vi "ID MDP RAZDTC.vi"(8 "errin":errorcluster) -> (0 "errout":errorcluster, 1 "snif can":string, 2 "Messout 3":T1 {"ID" format="%x"; "MSGTYPE" format="%.0x"; "LEN" format="%.0x"; "DATA[0]" format="%.0x"; "DATA[1]" format="%.0x"; "DATA[2]" format="%.0x"; "DATA[3]" format="%.0x"; "DATA[4]" format="%.0x"; "DATA[5]" format="%.0x"; "DATA[6]" format="%.0x"; "DATA[7]" format="%.0x"}, 3 "MSG":string)   [LabVIEW 2020]
uses:
  C/Program Files (x86)/National Instruments/LabVIEW 2020/user.lib/PCAN Basic/Controls/Channel.ctl
  C/Program Files (x86)/National Instruments/LabVIEW 2020/user.lib/PCAN Basic/Controls/BaudrateEenum.ctl
  C/Program Files (x86)/National Instruments/LabVIEW 2020/user.lib/PCAN Basic/PCANBasic.lvlib
  FGV.ctl
  C/Program Files (x86)/National Instruments/LabVIEW 2020/user.lib/Alex_Peak_lib/PEAK_lib_ALEX.lvlib
panel:
  out "EXIT":bool
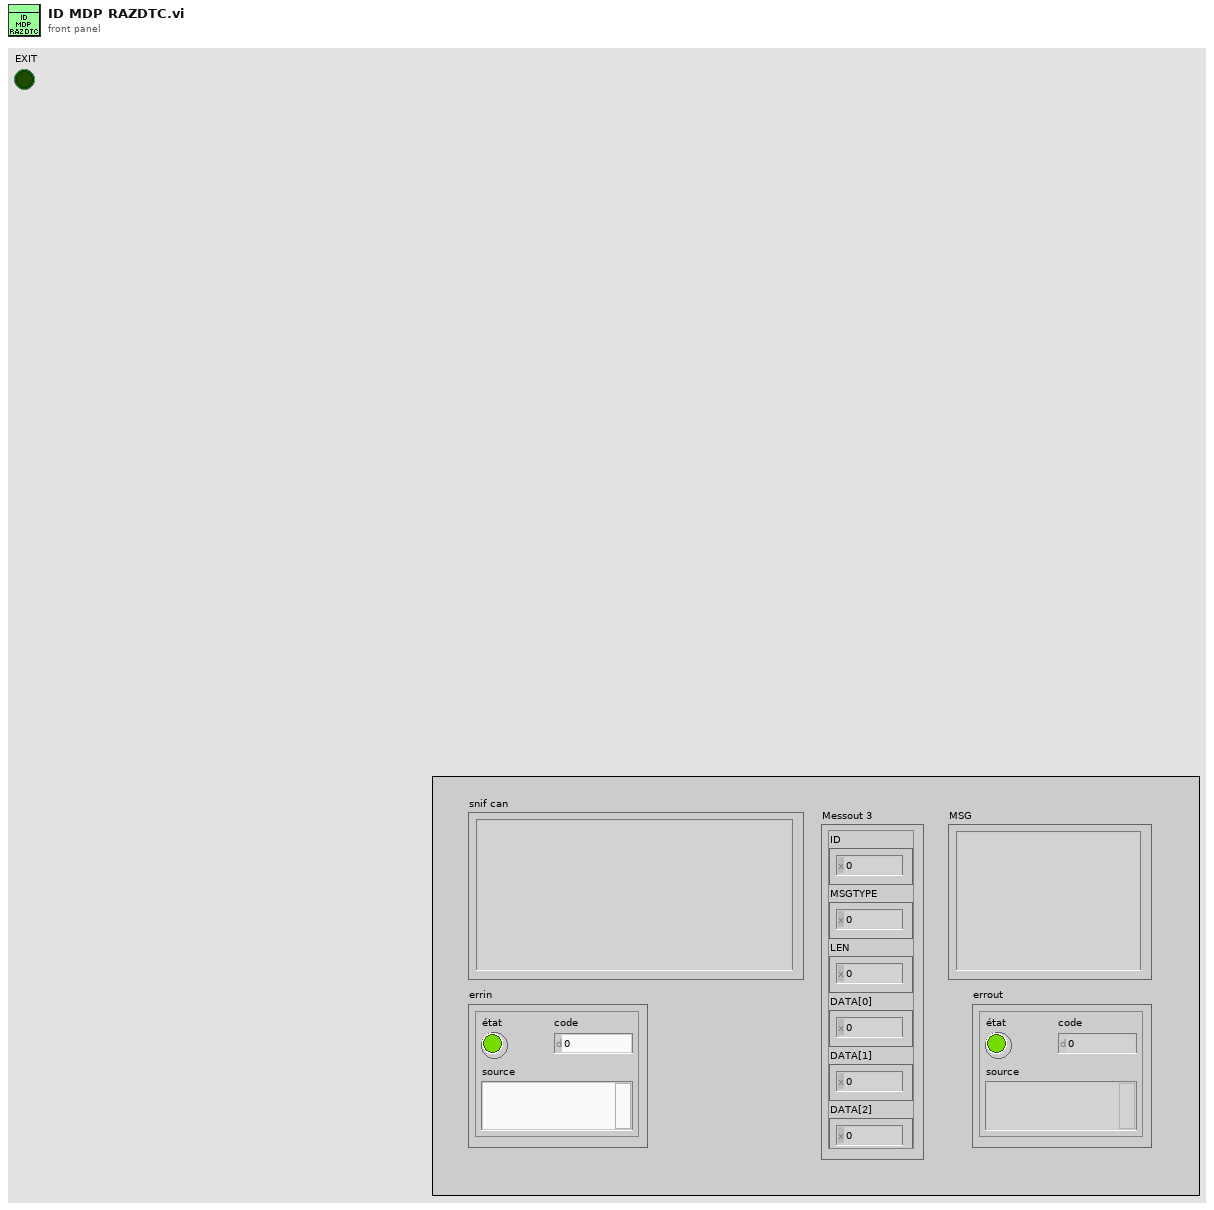
[diagram p1: front panel]
types:
  T1 = cluster{"ID":u32, "MSGTYPE":u8, "LEN":u8, "DATA[0]":u8, "DATA[1]":u8, "DATA[2]":u8, "DATA[3]":u8, "DATA[4]":u8, "DATA[5]":u8, "DATA[6]":u8, "DATA[7]":u8}
  T2 = typedef "PCANBasic.lvlib/BaudrateEenum.ctl" = enum16{"CAN_Baud_1M", "CAN_Baud_800K", "CAN_BAUD_500K", "CAN_BAUD_250K", "CAN_BAUD_125K", "CAN_BAUD_100K", "CAN_BAUD_95K", "CAN_BAUD_83K", "CAN_BAUD_50K", "CAN_BAUD_47K", "CAN_BAUD_33K", "CAN_BAUD_20K", "CAN_BAUD_10K", "CAN_BAUD_5K", "User Baudrate"}
  T3 = typedef "PCANBasic.lvlib/Channel.ctl" = enum16{"PCAN_NONEBUS", "not used1", "not used2", "not used3", "not used4", "not used5", "not used6", "not used7", "not used8", "not used9", "not used10", "not used11", "not used12", "not used13", "not used14", "not used15", "not used16", "not used17", "not used18", "not used19", "not used20", "not used21", "not used22", "not used23", "not used24", "not used25", "not used26", "not used27", "not used28", "not used29", "not used30", "not used31", "not used32", "PCAN_ISABUS1", "PCAN_ISABUS2", "PCAN_ISABUS3", "PCAN_ISABUS4", "PCAN_ISABUS5", "PCAN_ISABUS6", "PCAN_ISABUS7", "PCAN_ISABUS8", "not used41", "not used42", "not used43", "not used44", "not used45", "not used46", "not used47", "not used48", "PCAN_DNGBUS1", "not used50", "not used51", "not used52", "not used53", "not used54", "not used55", "not used56", "not used57", "not used58", "not used59", "not used60", "not used61", "not used62", "not used63", "not used64", "PCAN_PCIBUS1", "PCAN_PCIBUS2", "PCAN_PCIBUS3", "PCAN_PCIBUS4", "PCAN_PCIBUS5", "PCAN_PCIBUS6", "PCAN_PCIBUS7", "PCAN_PCIBUS8", "not used73", "not used74", "not used75", "not used76", "not used77", "not used78", "not used79", "not used80", "PCAN_USBBUS1", "PCAN_USBBUS2", "PCAN_USBBUS3", "PCAN_USBBUS4", "PCAN_USBBUS5", "PCAN_USBBUS6", "PCAN_USBBUS7", "PCAN_USBBUS8", "Not used89", "Not used90", "Not used91", "Not used92", "Not used93", "Not used94", "Not used95", "Not used96", "PCAN_PCCBUS1", "PCAN_PCCBUS2"}
  T4 = typedef "FGV.ctl" = enum16{"GET", "SET", "RAZ"}
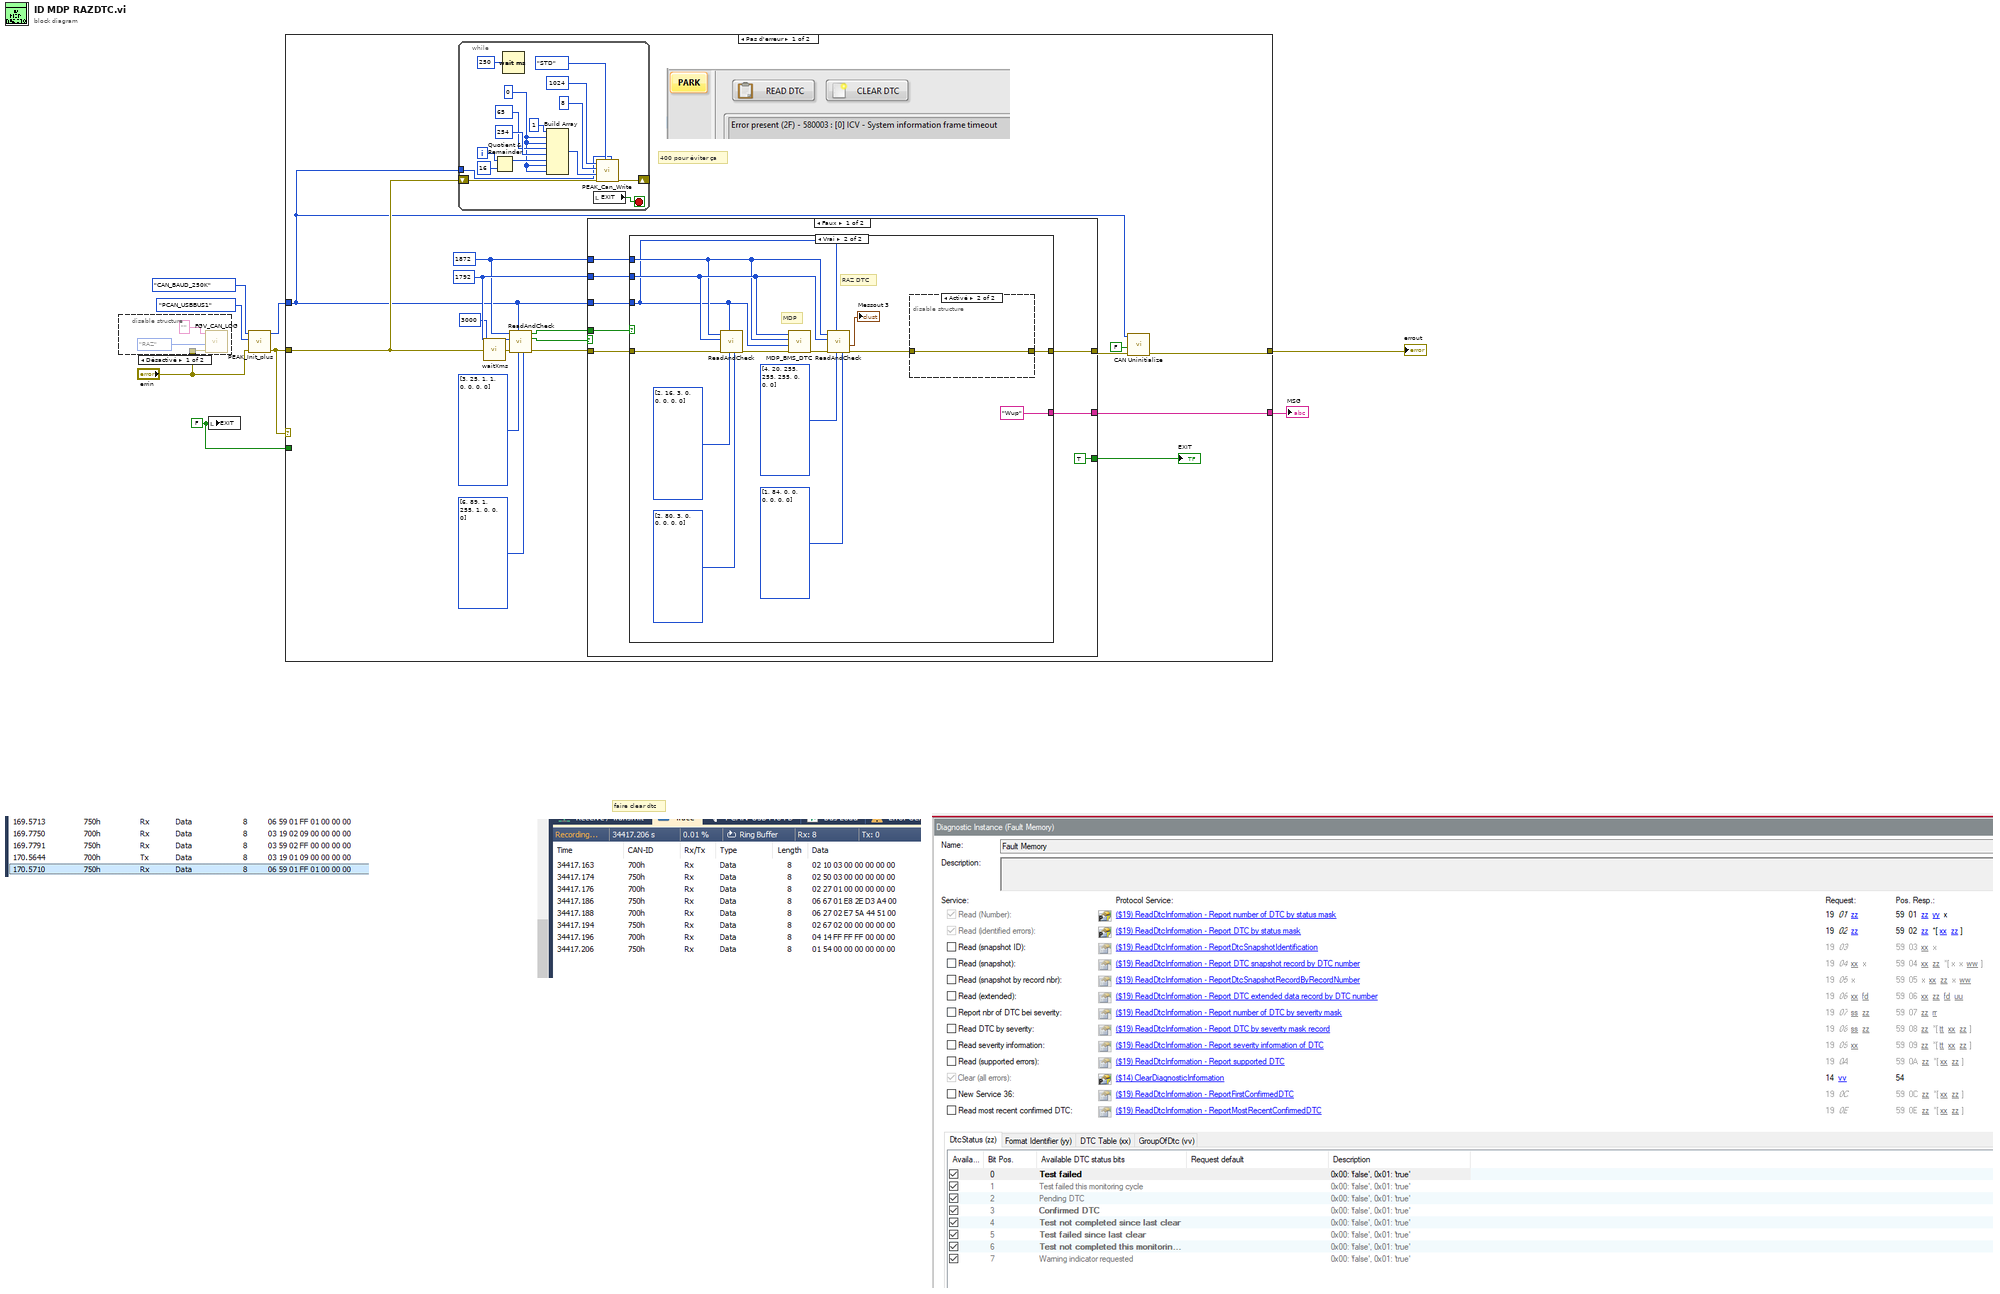
[diagram p0: block diagram]
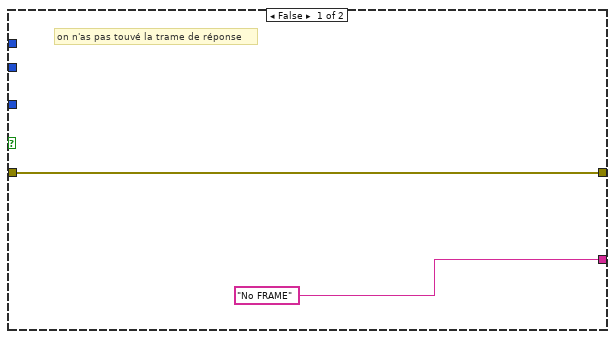
[diagram p3: hidden frame]
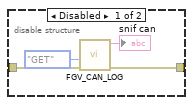
[diagram p4: hidden frame]
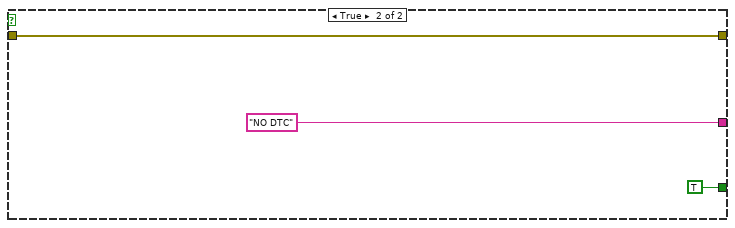
[diagram p5: hidden frame]
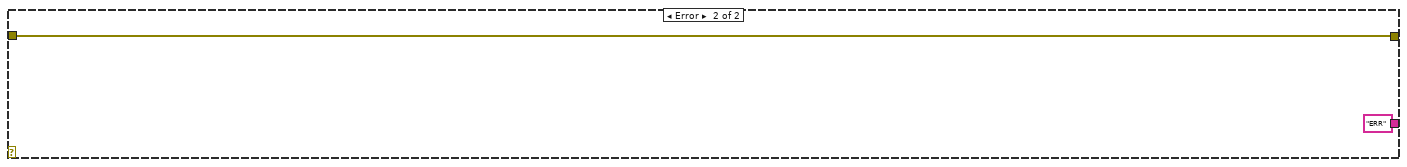
[diagram p6: hidden frame]
diagram:
  w3 = FALSE ("EXIT")
  # "faire clear dtc"
  n1 = disable-structure shown="Désactivé" {
    disable-tunnel: "errin" -> [w9 _]
    frame Disabled {
      n2 = call "FGV_CAN_LOG.vi"("errin"=w9, "CMD"=FGV."RAZ", "ChaineIn"="") -> ()  [unwired: 7 in, 2 out]
    }
    frame Enabled {
    }
  }
  n3 = local write "EXIT"(w3) -> ()
  n4 = call "PEAK_Init_plus.vi"("errin"="errin", "Channel"=Channel."PCAN_USBBUS1", "BTR0BTR1"=BaudrateEenum."CAN_BAUD_250K") -> ("errout"=w4:errorcluster, "Channel out"=w8:T3)  [unwired: 7 in]
  n5 = case shown="Pas d'erreur" w4 {
    tunnel: w8 -> [w14 _]
    tunnel: [w13 w77] -> w2
    tunnel: w4 -> [w17 w77]
    tunnel: [w20 "ERR" ("message")] -> w5
    tunnel: w3 -> [_ _]
    frame No Error {
      w25 = u32 1872 ("Identifier")
      w26 = u32 1792 ("Identifier")
      # "400 pour éviter ça"
      n6 = while {
        tunnel: w14 -> [w36]
        shift-right: [w43] -> _
        shift-left: w17 -> [w31]
        i -> [w35]
        stop <- w32 stop-if-true
        w28 = u8 0 ("élément")
        n7 = Quotient & Remainder(x=w35, y=16) -> (x-y*floor(x/y)=w33:i32)  [unwired: 1 out]
        n8 = Wait (ms)(milliseconds to wait=u32 250 ("attente (ms)")) -> ()  [unwired: 1 out]
        n9 = Build Array(1 ("élément"), w28, w28, u8 65 ("élément"), u8 254 ("élément"), w33, w28, w28) -> (w40:i32[])
        n10 = local read "EXIT"() -> (w32:bool)
        n11 = call "PEAK_Can_Write.vi"("CAN Handle"=w36, "MSG type"=enum8{"STD", "RTR", "XTD", "XTD RTR", "STATUS"}."STD", "errin"=w31, "CAN Data"=w40, "DLC (8)"=u8 8, "Identifier"=u32 1024) -> ("errout"=w43:errorcluster)  [unwired: 5 in]
      }
      n12 = call "waitXms.vi"("attente (ms)"=u32 3000, "errin"=w17) -> ("errout"=w19:errorcluster)  [unwired: 13 in]
      n13 = call "ReadAndCheck.vi"("GET"=u8[] [6, 89, 1, 255, 1, 0, 0, 0] ("y"), "SET"=u8[] [3, 25, 1, 1, 0, 0, 0, 0] ("y"), "ChanelIn"=w14, "errin"=w19, "TA"=w26, "SA"=w25) -> ("errout"=w27:errorcluster, "Identique"=w22:bool, "trouvé"=w21:bool)  [unwired: 2 in, 1 out]
      n14 = case shown="Faux" w22 {
        tunnel: [w51 w75] -> w15
        tunnel: w27 -> [w50 w75]
        tunnel: w26 -> [w49 _]
        tunnel: w25 -> [w48 _]
        tunnel: w14 -> [w47 _]
        tunnel: w21 -> [w46 _]
        tunnel: [w45 "NO DTC" ("message")] -> w20
        tunnel: [TRUE TRUE] -> w16
        frame False {
          n15 = case shown="Vrai" w46 {
            tunnel: [w53 w59] -> w51
            tunnel: w50 -> [w53 w58]
            tunnel: w49 -> [_ w57]
            tunnel: w48 -> [_ w56]
            tunnel: w47 -> [_ w55]
            tunnel: ["No FRAME" ("message") "Wup" ("message")] -> w45
            frame False {
              # "on n'as pas touvé la trame de réponse"
            }
            frame True {
              # "RAZ DTC"
              # "MDP"
              n16 = call "ReadAndCheck.vi"("GET"=u8[] [2, 80, 3, 0, 0, 0, 0, 0] ("y"), "SET"=u8[] [2, 16, 3, 0, 0, 0, 0, 0] ("y"), "ChanelIn"=w55, "errin"=w58, "TA"=w57, "SA"=w56) -> ("errout"=w63:errorcluster)  [unwired: 2 in, 3 out]
              n17 = call "MDP_BMS_DTC.vi"("errin"=w63, "Channel out"=w55, "SA"=w56, "TA"=w57) -> ("errout"=w64:errorcluster)  [unwired: 6 in, 1 out]
              n18 = call "ReadAndCheck.vi"("GET"=u8[] [1, 84, 0, 0, 0, 0, 0, 0] ("y"), "SET"=u8[] [4, 20, 255, 255, 255, 0, 0, 0] ("y"), "ChanelIn"=w55, "errin"=w64, "TA"=w57, "SA"=w56) -> ("errout"=w60:errorcluster, "Messout"=→"Messout 3":T1)  [unwired: 2 in, 2 out]
              n19 = disable-structure shown="Activé" {
                disable-tunnel: w60 -> [w71 w72]
                disable-tunnel: [w70 w72] -> w59
                frame Disabled {
                  n20 = call "FGV_CAN_LOG.vi"("errin"=w71, "CMD"=FGV."GET") -> ("errout"=w70:errorcluster, "Chaîne"=→"snif can":string)  [unwired: 8 in]
                }
                frame Enabled {
                }
              }
            }
          }
        }
        frame True {
        }
      }
      "EXIT" <- w16
      n21 = call "CAN Uninitialize.vi"("error in (no error)"=w15, "Ignore input error"=FALSE, "Channel"=w14) -> ("error out"=w13:errorcluster)  [unwired: 6 in, 2 out]
    }
    frame Error {
    }
  }
  "errout" <- w2
  "MSG" <- w5
